vi "Channel Count (Plugin).vi"(8 "error in (no error)":errorcluster, 11 "Plugin Configuration in":T1={"name"="", "components"=[], "cycle timing"={"priority"=0, "decimation"=1, "offset"=0}, "threads"=[], "transfer groups"=[], "settings"=[]} {"transfer groups"."transfers"."channels"."string offset" format="%d bytes"}) -> (0 "error out":errorcluster, 2 "total channel count":u64, 3 "Plugin Configuration out":T1={"name"="", "components"=[], "cycle timing"={"priority"=0, "decimation"=1, "offset"=0}, "threads"=[], "transfer groups"=[], "settings"=[]} {"transfer groups"."transfers"."channels"."string offset" format="%d bytes"})   [LabVIEW 2017, in "DSF Core.lvlib" / "Configuration Session.lvclass"]
uses:
  Configuration Session.lvclass
  Typedefs/DSF Engine Plugin Configuration.ctl
  Typedefs/DSF Timing Info.ctl
  Typedefs/DSF Engine Plugin Thread Configuration.ctl
  Typedefs/DSF Settings Info.ctl
  Typedefs/DSF Engine Transfer Group Configuration.ctl
  Typedefs/DSF Direction.ctl
  Typedefs/DSF Engine Transfer Configuration.ctl
  Typedefs/DSF Byte Order.ctl
  Typedefs/DSF Engine Channel Configuration.ctl
  Typedefs/DSF Data Type.ctl
  Typedefs/DSF Timeout Behavior.ctl
  DSF Core.lvlib
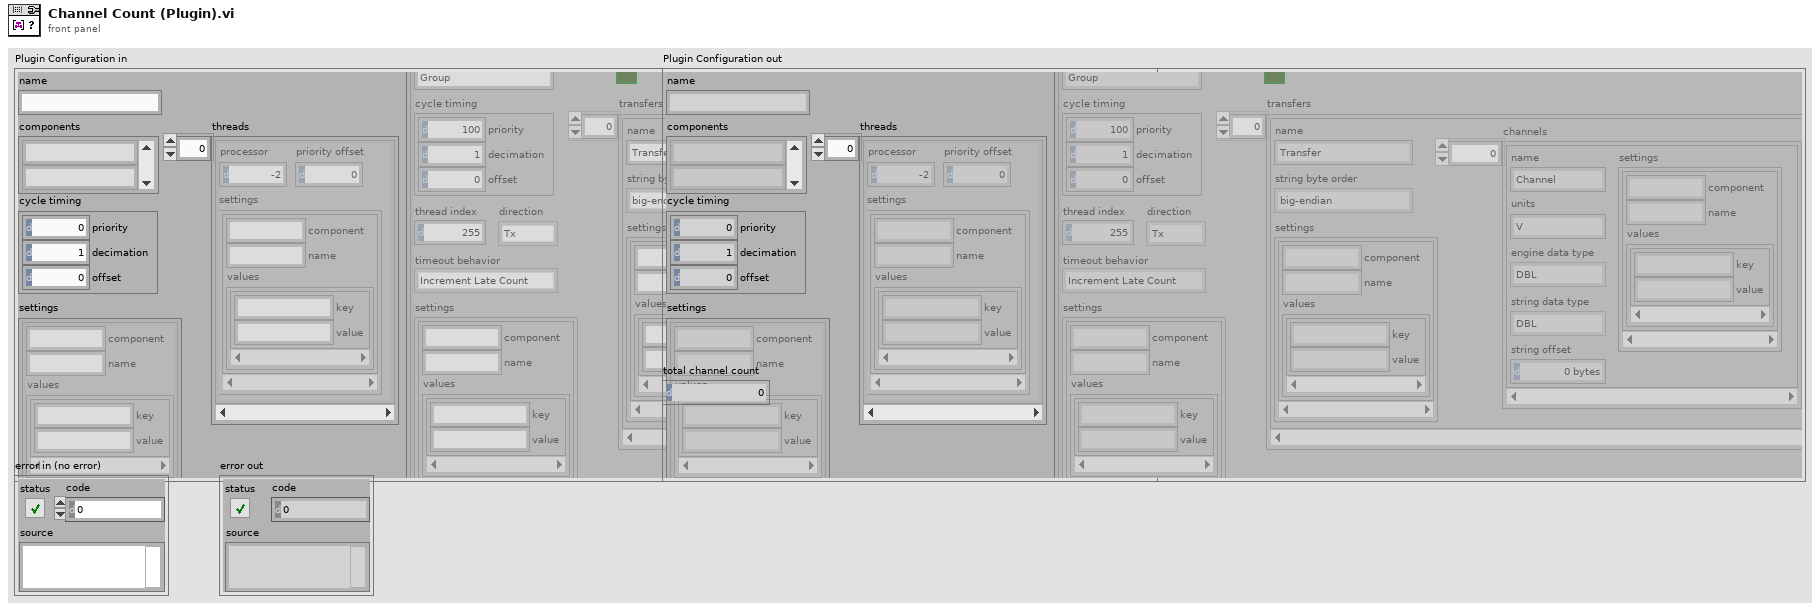
[diagram p1: front panel]
types:
  T1 = typedef "DSF Core.lvlib/DSF Engine Plugin Configuration.ctl" = cluster{"name":string, "components":string[], "cycle timing":T2, "threads":T3[], "transfer groups":T5[], "settings":T4}
  T2 = typedef "DSF Core.lvlib/DSF Timing Info.ctl" = cluster{"priority":u64, "decimation":u64, "offset":u64}
  T3 = typedef "DSF Core.lvlib/DSF Engine Plugin Thread Configuration.ctl" = cluster{"processor":i32, "priority offset":i16, "settings":T4}
  T4 = typedef "DSF Core.lvlib/DSF Settings Info.ctl" = cluster{"component":string, "name":string, "values":cluster{"key":string, "value":string}[]}[]
  T5 = typedef "DSF Core.lvlib/DSF Engine Transfer Group Configuration.ctl" = cluster{"name":string, "direction":T6, "cycle timing":T2, "thread index":u8, "settings":T4, "transfers":T7[], "timeout behavior":T11, "convert buffers":bool}
  T6 = typedef "DSF Core.lvlib/DSF Direction.ctl" = enum8{"Tx", "Rx"}
  T7 = typedef "DSF Core.lvlib/DSF Engine Transfer Configuration.ctl" = cluster{"name":string, "string byte order":T8, "settings":T4, "channels":T9[]}
  T8 = typedef "DSF Core.lvlib/DSF Byte Order.ctl" = enum8{"big-endian", "little-endian"}
  T9 = typedef "DSF Core.lvlib/DSF Engine Channel Configuration.ctl" = cluster{"string offset":u64, "name":string, "units":string, "engine data type":T10, "string data type":T10, "settings":T4}
  T10 = typedef "DSF Core.lvlib/DSF Data Type.ctl" = enum8{"Bool", "SGL", "DBL", "I8", "I16", "I32", "I64", "U8", "U16", "U32", "U64"}
  T11 = typedef "DSF Core.lvlib/DSF Timeout Behavior.ctl" = enum8{"Increment Late Count", "Throw Error"}
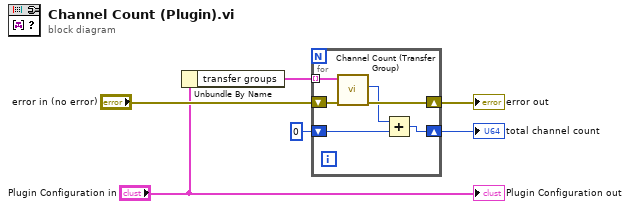
[diagram p0: block diagram]
diagram:
  n1 = Unbundle By Name("Plugin Configuration in") -> ("transfer groups"=w4:T5[])
  n2 = for {
    tunnel: w4 -> [w10] mode=indexing
    shift-right: [w12] -> w5
    shift-left: u64 0 -> [w11]
    shift-right: [w8] -> w3
    shift-left: "error in (no error)" -> [w9]
    n3 = call "Channel Count (Transfer Group).vi"("error in (no error)"=w9, "Transfer Group Configuration in"=w10) -> ("error out"=w8:errorcluster, "total channel count"=w7:u64)  [unwired: 7 in, 1 out]
    n4 = Add(x=w7, y=w11) -> (x+y=w12:u64)
  }
  "total channel count" <- w5
  "error out" <- w3
  "Plugin Configuration out" <- "Plugin Configuration in"
